vi "DLIWebPowerSwitch.vi"(4 "Scan Period":dbl format="%.2f", 5 "Previous Scan Value":dbl format="%.2f", 6 "Present scan array":dbl[](array[numeric]) format="%.2f", 7 "Value to Output":dbl format="%.2f", 8 "Ch Description":T1={"Ch Name"="Valve8", "Type"="DLI WebPowerSwitch", "Function"=enum."Relay Output", "Ch State"=enum."On", "Calibration type"=enum."Raw", "A"=200.0, "B"=0.0, "C"=0.0, "D"=0.0, "Comments"="", "Address"={"Main"=0, "Ch."=1, "Sub"=0, "Port Name"="192.168.126.155"}, "String"="LV:LV", "Duty"=65535} {"Duty" format="%016b"; "D" format="%#_5g"; "C" format="%#_5g"; "B" format="%#_5g"; "A" format="%#_5g"}, 9 "Ch names":string[](array[string])) -> (0 "Scan comment":string, 1 "Output":dbl format="%.3f", 3 "HelpText":string="Value to Output: 1-On 0-Off 99-Toggle\nOutput state is read back, and will be 0 for Off, 1 for On\n\"Port Name\" contains the IP address of the unit\nCh. is used to specify the outlet number, 1-8\nComment (the red box) is used for username:password\n\"A\" is the timeout, in ms")   [LabVIEW 2016]
uses:
  ADAM Client/Sub VIs/ADAM Controls/Ch_description_ADAM.ctl
  ADAM Client/Sub VIs/ADAM Controls/Module_type_ADAM.ctl
  ADAM Client/Sub VIs/ADAM Controls/Function_ADAM.ctl
  ADAM Client/Sub VIs/ADAM Controls/Channel_State.ctl
  ADAM Client/Sub VIs/ADAM Controls/Calib_type_ADAM.ctl
  ADAM Client/Sub VIs/ADAM Controls/Address.ctl
  <vilib>/Utility/error.llb/DialogType.ctl
  <vilib>/httpClient/LabVIEWHTTPClient.lvlib
panel:
  out "body":string
  out "headers":string
  # "VI to control the Digital Loggers International Web Power Switch"
  # "https://www.digital-loggers.com/lpc.html"
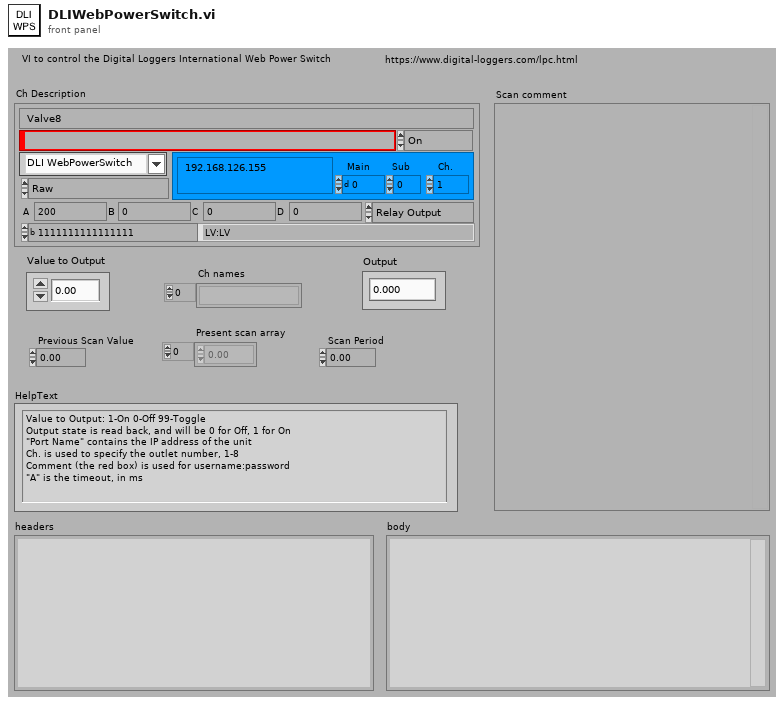
[diagram p1: front panel]
types:
  T1 = typedef "Ch_description_ADAM.ctl" = cluster{"Ch Name":string, "Type":T2, "Function":T3, "Ch State":T4, "Calibration type":T5, "A":dbl, "B":dbl, "C":dbl, "D":dbl, "Comments":string, "Address":T6, "String":string, "Duty":u16}
  T2 = typedef "Module_type_ADAM.ctl" = string
  T3 = typedef "Function_ADAM.ctl" = enum16{"Analogue Input", "Digital Input", "Event counter", "Event rate", "Analogue Output", "Digital Output", "Relay Output"}
  T4 = typedef "Channel_State.ctl" = enum16{"On", "Off", "Always On", "Always Off"}
  T5 = typedef "Calib_type_ADAM.ctl" = enum16{"Raw", "Bx + A", "Cx^2 + Bx + A", "Dx^3 + Cx^2 + Bx + A", "In Band", "Hi-Tec Q", "Hi-Tec M_dot", "Text"}
  T6 = typedef "Address.ctl" = cluster{"Main":i32, "Ch.":i32, "Sub":i32, "Port Name":string}
  T7 = typedef "DialogType.ctl" = u16
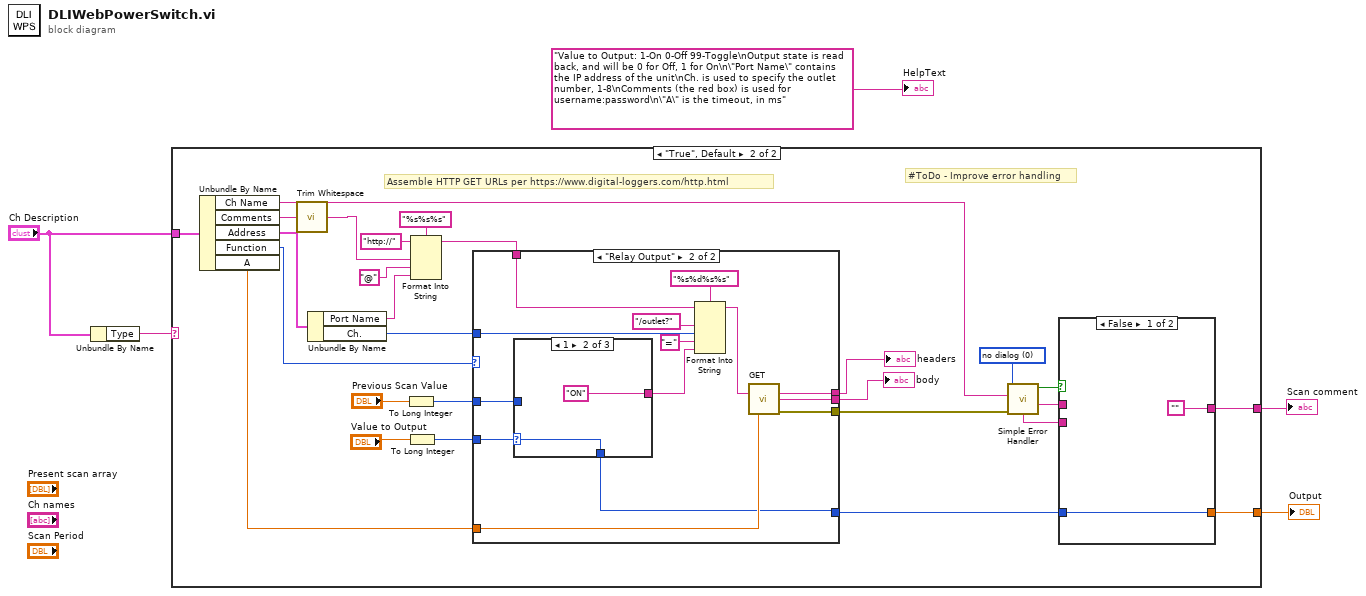
[diagram p0: block diagram]
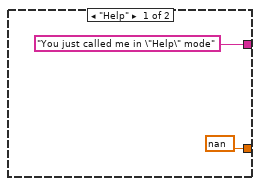
[diagram p2: hidden frame]
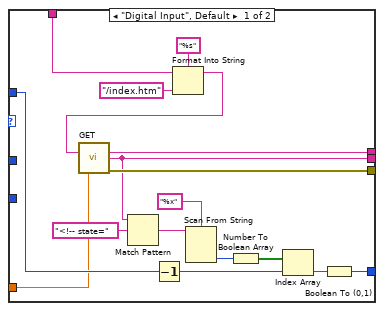
[diagram p3: hidden frame]
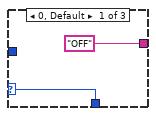
[diagram p4: hidden frame]
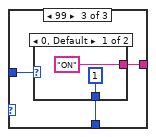
[diagram p5: hidden frame]
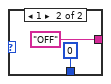
[diagram p6: hidden frame]
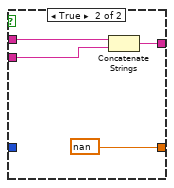
[diagram p7: hidden frame]
diagram:
  n1 = Unbundle By Name("Ch Description") -> ("Type"=w2:T2)
  n2 = case shown="\"True\", Default" w2 {
    tunnel: ["You just called me in \"Help\" mode" w29] -> w5
    tunnel: [nan ("t") w28] -> w4
    tunnel: "Ch Description" -> [_ w20]
    frame "Help" {
    }
    frame "True", Default {
      w34 = T7 0 items=["no dialog", "OK message", "continue or stop message", "OK message + warnings", "continue/stop + warnings"] ("type of dialog (OK msg:1)")
      # "#ToDo - Improve error handling"
      # "Assemble HTTP GET URLs per https://www.digital-loggers.com/http.html"
      n3 = Unbundle By Name(w20) -> ("Ch Name"=w21:string, "Comments"=w9:string, "Address"=w31:T6, "Function"=w17:T3, "A"=w14:dbl)
      n4 = call <vilib>:"Trim Whitespace.vi"("string"=w9) -> ("trimmed string"=w8:string)  [unwired: 1 in]
      n5 = Unbundle By Name(w31) -> ("Port Name"=w25:string, "Ch."=w22:i32)
      n6 = To Long Integer(number="Previous Scan Value") -> (32bit integer=w10:i32)
      n7 = To Long Integer(number="Value to Output") -> (32bit integer=w11:i32)
      n8 = Format Into String(format string="%s%s%s", initial string="http://", w8, "@" ("input 2"), w25) -> (resulting string=w23:string)  [unwired: 1 in, 1 out]
      n9 = case shown="\"Relay Output\"" w17 {
        tunnel: [w40 w61] -> w16
        tunnel: w23 -> [w41 w60]
        tunnel: w22 -> [w39 w59]
        tunnel: w14 -> [w38 w56]
        tunnel: [w36 w58] -> w19
        tunnel: [w37 w57] -> w18
        tunnel: [w35 w54] -> w15
        tunnel: w11 -> [_ w53]
        tunnel: w10 -> [_ w52]
        frame "Digital Input", Default {
          n10 = Decrement(x=w39) -> (x-1=w50:i32)
          n11 = Format Into String(format string="%s", initial string=w41, "/index.htm" ("input 1")) -> (resulting string=w43:string)  [unwired: 1 in, 1 out]
          n12 = call <vilib>:"GET.vi"("url"=w43, "timeout (10000)"=w38) -> ("headers"=w36:string, "body"=w37:string, "error out"=w40:errorcluster)  [unwired: 10 in, 1 out]
          n13 = Match Pattern(string=w37, regular expression="<!-- state=") -> (after substring=w46:string)  [unwired: 1 in, 3 out]
          n14 = Scan From String(format string="%x", input string=w46) -> (output 1=w48:u32)  [unwired: 3 in, 3 out]
          n15 = Number To Boolean Array(number=w48) -> (Boolean array=w49:bool[])
          n16 = Index Array(array=w49, index=w50) -> (element=w51:bool)
          n17 = Boolean To (0,1)(Boolean=w51) -> (0, 1=w35:i16)
        }
        frame "Relay Output" {
          n18 = case shown="1" w53 {
            selector: w53 -> [w66 w68 _]
            tunnel: ["OFF" "ON" w72] -> w55
            tunnel: [w66 w68 w71] -> w54
            tunnel: w52 -> [_ _ w70]
            frame 0, Default {
            }
            frame 1 {
            }
            frame 99 {
              n19 = case shown="0, Default" w70 {
                tunnel: ["ON" "OFF"] -> w72
                tunnel: [i16 1 i16 0] -> w71
                frame 0, Default {
                }
                frame 1 {
                }
              }
            }
          }
          n20 = Format Into String(format string="%s%d%s%s", initial string=w60, "/outlet?" ("input 4"), w59, "=", w55) -> (resulting string=w62:string)  [unwired: 1 in, 1 out]
          n21 = call <vilib>:"GET.vi"("url"=w62, "timeout (10000)"=w56) -> ("headers"=w58:string, "body"=w57:string, "error out"=w61:errorcluster)  [unwired: 10 in, 1 out]
        }
      }
      "headers" <- w19
      "body" <- w18
      n22 = call <vilib>:"Simple Error Handler.vi"("error source (\" \")"=w21, "type of dialog (OK msg:1)"=w34, "error in (no error)"=w16) -> ("error?"=w30:bool, "source out"=w32:string, "message"=w33:string)  [unwired: 4 out]
      n23 = case shown="False" w30 {
        tunnel: w33 -> [_ w80]
        tunnel: w32 -> [_ w81]
        tunnel: ["" w79] -> w29
        tunnel: [w77 nan ("t")] -> w28
        tunnel: w15 -> [w77 _]
        frame False {
        }
        frame True {
          n24 = Concatenate Strings(w81, w80) -> (w79:string)
        }
      }
    }
  }
  "Output" <- w4
  "Scan comment" <- w5
  "HelpText" <- "Value to Output: 1-On 0-Off 99-Toggle\nOutput state is read back, and will be 0 for Off, 1 for On\n\"Port Name\" contains the IP address of the unit\nCh. is used to specify the outlet number, 1-8\nComments (the red box) is used for username:password\n\"A\" is the timeout, in ms"
